vi "Is Cell a Date.vi"(8 "error in":errorcluster, 10 "Cell in":refnum<k24>, 11 "SpreadsheetDoc in":refnum<k24>) -> (0 "error out":errorcluster, 1 "Is Date":bool, 2 "Cell out":refnum<k24>, 3 "SpreadsheetDoc out":refnum<k24>)   [LabVIEW 2019, in "Open Xml.lvlib"]
uses:
  Open Xml.lvlib
  D:/git/Open-Xml-LabVIEW/Source/DocumentFormat.OpenXml.dll
  DocumentFormat.OpenXml.dll
  D:/git/Open-Xml-LabVIEW/Source/DocumentFormat.OpenXml.Framework.dll
  DocumentFormat.OpenXml.Framework.dll
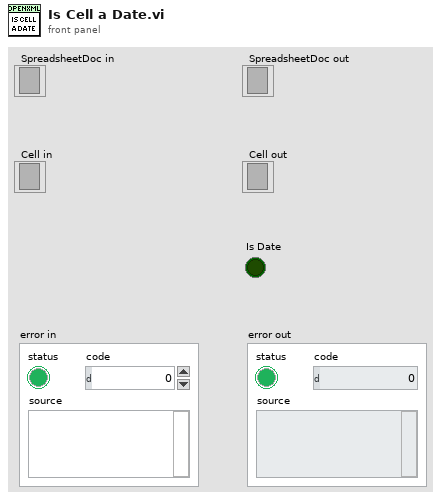
[diagram p1: front panel]
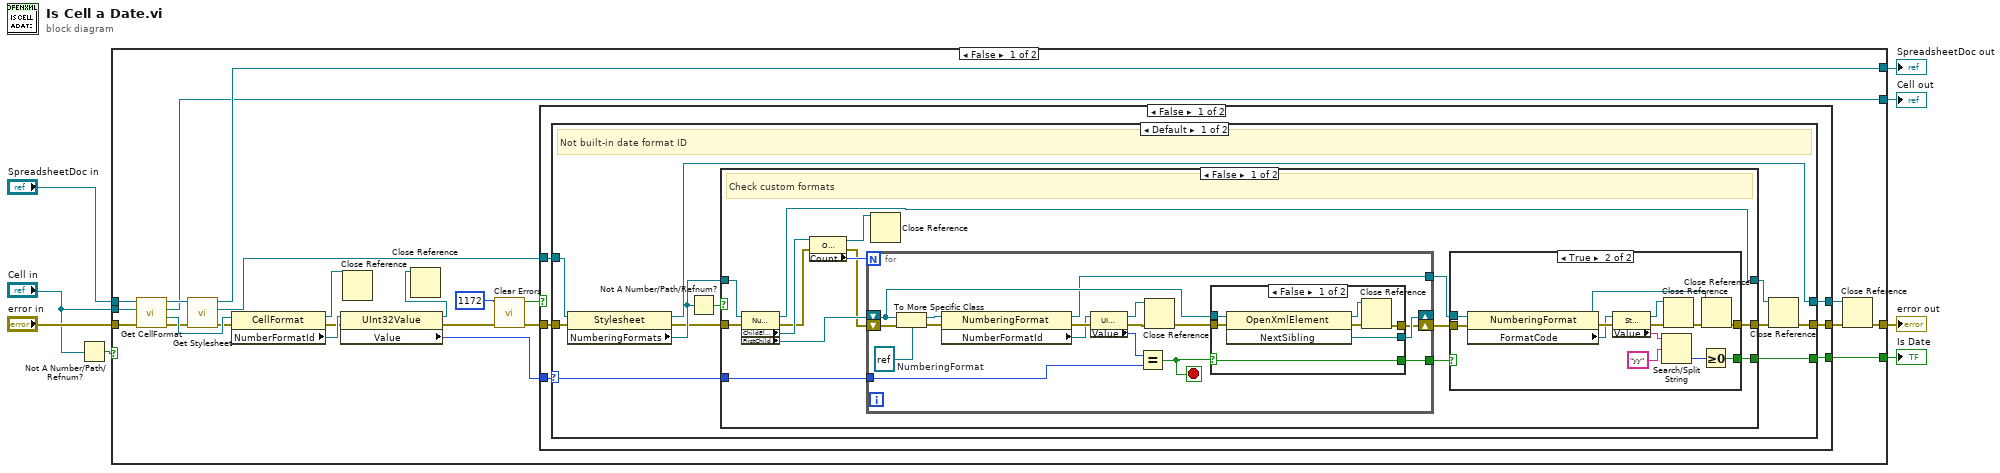
[diagram p0: block diagram]
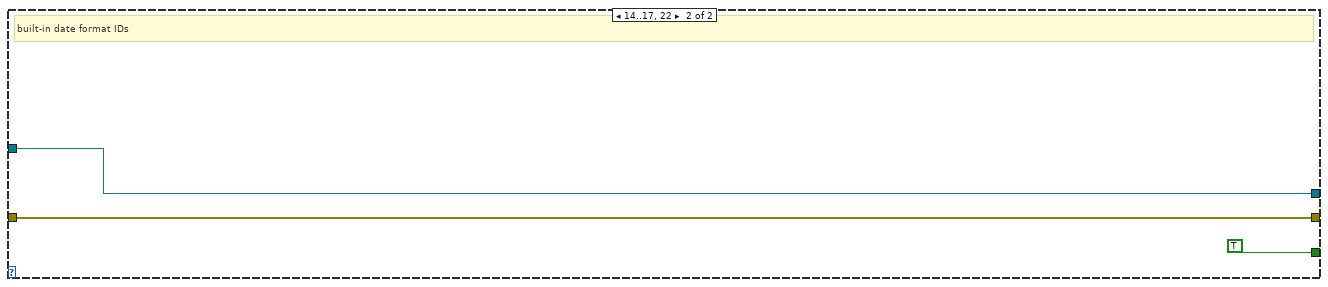
[diagram p5: hidden frame]
diagram:
  n1 = Not A Number/Path/Refnum?(number/path/refnum="Cell in") -> (NaN/Path/Refnum?=w6:bool)
  n2 = case shown="False" w6 {
    tunnel: "error in" -> [w30 w113]
    tunnel: [w26 _] -> w7
    tunnel: "Cell in" -> [w21 w112]
    tunnel: "SpreadsheetDoc in" -> [w31 w114]
    tunnel: [w18 w114] -> w4
    tunnel: [w13 w113] -> w3
    tunnel: [w15 w112] -> w1
    frame False {
      n3 = call "Get CellFormat.vi"("error in"=w30, "Cell In"=w21, "SpreadsheetDoc in"=w31) -> ("error out"=w16:errorcluster, "CellFormat"=w29:refnum<k24>, "Cell out"=w15:refnum<k24>, "SpreadsheetDoc out"=w19:refnum<k24>)  [unwired: 5 in]
      n4 = call "Get Stylesheet.vi"("error in"=w16, "SpreadsheetDoc in"=w19) -> ("error out"=w20:errorcluster, "Stylesheet"=w17:refnum<k24>, "SpreadsheetDoc out"=w18:refnum<k24>)  [unwired: 7 in]
      n5 = property class="CellFormat"(reference=w29, error in=w20) -> (reference out=w23:refnum<k24>, error out=w25:errorcluster, "NumberFormatId"=w28:refnum<k24>)
      n6 = property class="UInt32Value"(reference=w28, error in=w25) -> (reference out=w24:refnum<k24>, error out=w14:errorcluster, "Value"=w27:u32)
      n7 = Close Reference(reference=w23) -> ()  [unwired: 1 in, 1 out]
      n8 = Close Reference(reference=w24) -> ()  [unwired: 1 in, 1 out]
      n9 = call <vilib>:"Clear Errors.vi"("error in (no error)"=w14, "specific error code to clear (0: all)"=1172) -> ("error out"=w11:errorcluster, "specific error cleared?"=w9:bool)  [unwired: 4 in]
      n10 = case shown="False" w9 {
        tunnel: w27 -> [w37 _]
        tunnel: [w36 _] -> w26
        tunnel: [w35 w111] -> w22
        tunnel: w17 -> [w34 w110]
        tunnel: [w33 w110] -> w12
        tunnel: w11 -> [w32 w111]
        frame False {
          n11 = case shown="Default" w37 {
            selector: w37 -> [w44 _]
            tunnel: [w46 TRUE] -> w36
            tunnel: w32 -> [w41 w108]
            tunnel: w34 -> [w48 w107]
            tunnel: [w39 w108] -> w35
            tunnel: [w40 w107] -> w33
            frame Default {
              # "Not built-in date format ID"
              n12 = property class="Stylesheet"(reference=w48, error in=w41) -> (reference out=w40:refnum<k24>, error out=w42:errorcluster, "NumberingFormats"=w45:refnum<k24>)
              n13 = Not A Number/Path/Refnum?(number/path/refnum=w45) -> (NaN/Path/Refnum?=w47:bool)
              n14 = case shown="False" w47 {
                tunnel: [w55 _] -> w46
                tunnel: w45 -> [w63 w105]
                tunnel: w44 -> [w57 _]
                tunnel: [w51 w106] -> w43
                tunnel: w42 -> [w52 w106]
                tunnel: [w49 w105] -> w38
                frame False {
                  # "Check custom formats"
                  n15 = property class="NumberingFormats"(reference=w63, error in=w52) -> (reference out=w49:refnum<k24>, error out=w60:errorcluster, "ChildElements"=w62:refnum<k24>, "FirstChild"=w59:refnum<k24>)
                  n16 = property class="OpenXmlElementList"(reference=w62, error in=w60) -> (reference out=w50:refnum<k24>, error out=w58:errorcluster, "Count"=w61:i32)
                  n17 = for {
                    N: w61 -> [_]
                    shift-right: [w67] -> _
                    shift-left: w59 -> [w69]
                    shift-right: [w66] -> w54
                    shift-left: w58 -> [w79]
                    tunnel: w57 -> [w73]
                    tunnel: [w68] -> w56
                    tunnel: [w64] -> w53
                    stop <- w65 stop-if-true
                    w80 = refnum<k24> refnum  # NumberingFormat
                    n18 = To More Specific Class(target class=w80, reference=w69, error in=w79) -> (specific class reference=w78:refnum<k24>, error out=w77:errorcluster)
                    n19 = property class="NumberingFormat"(reference=w78, error in=w77) -> (reference out=w68:refnum<k24>, error out=w76:errorcluster, "NumberFormatId"=w75:refnum<k24>)
                    n20 = property class="UInt32Value"(reference=w75, error in=w76) -> (reference out=w72:refnum<k24>, error out=w71:errorcluster, "Value"=w74:u32)
                    n21 = Equal?(x=w74, y=w73) -> (x = y?=w65:bool)
                    n22 = Close Reference(reference=w72, error in (no error)=w71) -> (error out=w70:errorcluster)
                    n23 = case shown="False" w65 {
                      selector: w65 -> [w81 w90]
                      tunnel: w70 -> [w87 w89]
                      tunnel: w69 -> [w86 w88]
                      tunnel: [w85 w88] -> w67
                      tunnel: [w82 w89] -> w66
                      tunnel: [w81 w90] -> w64
                      frame False {
                        n24 = invoke class="OpenXmlElement" method="NextSibling"(reference=w86, error in=w87) -> (reference out=w84:refnum<k24>, error out=w83:errorcluster, "NextSibling"=w85:refnum<k24>)  [unwired: 1 in]
                        n25 = Close Reference(reference=w84, error in (no error)=w83) -> (error out=w82:errorcluster)
                      }
                      frame True {
                      }
                    }
                  }
                  n26 = Close Reference(reference=w50) -> ()  [unwired: 1 in, 1 out]
                  n27 = case shown="True" w53 {
                    tunnel: w56 -> [_ w104]
                    tunnel: [_ w98] -> w55
                    tunnel: [w91 w93] -> w51
                    tunnel: w54 -> [w91 w96]
                    frame False {
                    }
                    frame True {
                      n28 = property class="NumberingFormat"(reference=w104, error in=w96) -> (reference out=w92:refnum<k24>, error out=w103:errorcluster, "FormatCode"=w102:refnum<k24>)
                      n29 = property class="StringValue"(reference=w102, error in=w103) -> (reference out=w95:refnum<k24>, error out=w97:errorcluster, "Value"=w101:string)
                      n30 = Search/Split String(string=w101, search string/char (-)="yy") -> (offset of match=w99:i32)  [unwired: 1 in, 2 out]
                      n31 = Close Reference(reference=w95, error in (no error)=w97) -> (error out=w94:errorcluster)
                      n32 = Greater Or Equal To 0?(x=w99) -> (x >= 0?=w98:bool)
                      n33 = Close Reference(reference=w92, error in (no error)=w94) -> (error out=w93:errorcluster)
                    }
                  }
                }
                frame True {
                }
              }
              n34 = Close Reference(reference=w38, error in (no error)=w43) -> (error out=w39:errorcluster)
            }
            frame 14..17, 22 {
              # "built-in date format IDs"
            }
          }
        }
        frame True {
        }
      }
      n35 = Close Reference(reference=w12, error in (no error)=w22) -> (error out=w13:errorcluster)
    }
    frame True {
    }
  }
  "error out" <- w3
  "Is Date" <- w7
  "SpreadsheetDoc out" <- w4
  "Cell out" <- w1
